vi "Create unexist Folder.vi"(8 "error in (no error)":errorcluster, 11 "Path":path) -> (0 "error out":errorcluster, 3 "Path Out":path)   [LabVIEW 2017, in "File.lvlib"]
uses:
  File.lvlib
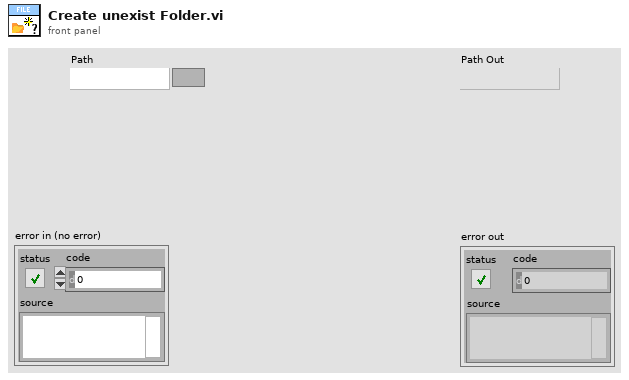
[diagram p1: front panel]
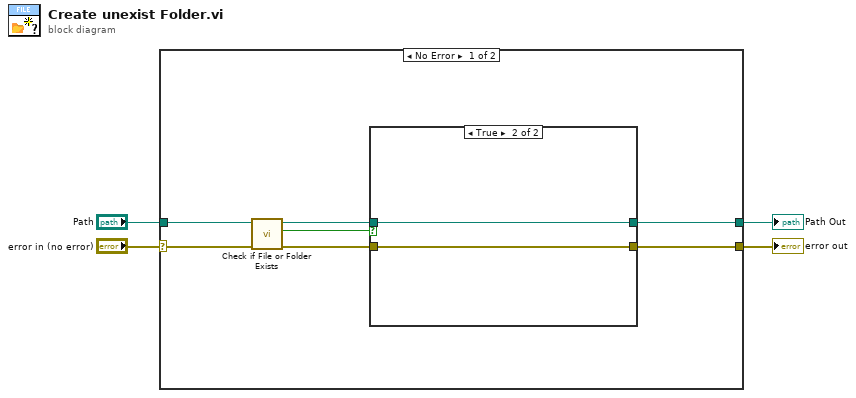
[diagram p0: block diagram]
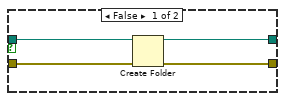
[diagram p2: hidden frame]
diagram:
  n1 = case shown="No Error" "error in (no error)" {
    selector: "error in (no error)" -> [w11 w19]
    tunnel: [w9 w19] -> w3
    tunnel: "Path" -> [w6 w18]
    tunnel: [w5 w18] -> w1
    frame No Error {
      n2 = call <vilib>:"Check if File or Folder Exists.vi"("error in (no error)"=w11, "path"=w6) -> ("error out"=w10:errorcluster, "file or folder exists?"=w8:bool, "dup path"=w7:path)  [unwired: 7 in]
      n3 = case shown="True" w8 {
        tunnel: w10 -> [w15 w17]
        tunnel: [w14 w17] -> w9
        tunnel: w7 -> [w13 w16]
        tunnel: [w12 w16] -> w5
        frame False {
          n4 = Create Folder(path (use dialog)=w13, error in=w15) -> (created path=w12:path, error out=w14:errorcluster)  [unwired: 1 in, 1 out]
        }
        frame True {
        }
      }
    }
    frame Error {
    }
  }
  "error out" <- w3
  "Path Out" <- w1
